vi "蝴蝶图 copy.vi"() -> ()   [LabVIEW 2023]
panel:
  out "XY Graph":cluster{"Y":dbl[], "Y":dbl[]}[](graph)
  out "return value":dbl[][](array[numeric])
  in  "Array 3":dbl[][](array[numeric])
  in  "module path 2":path
  out "error out 2":errorcluster
  out "error out":errorcluster
  in  "module path":path
  out "Array 2":string[](array[string])
  in  "String":string
  in  "Array":string[](array[string])
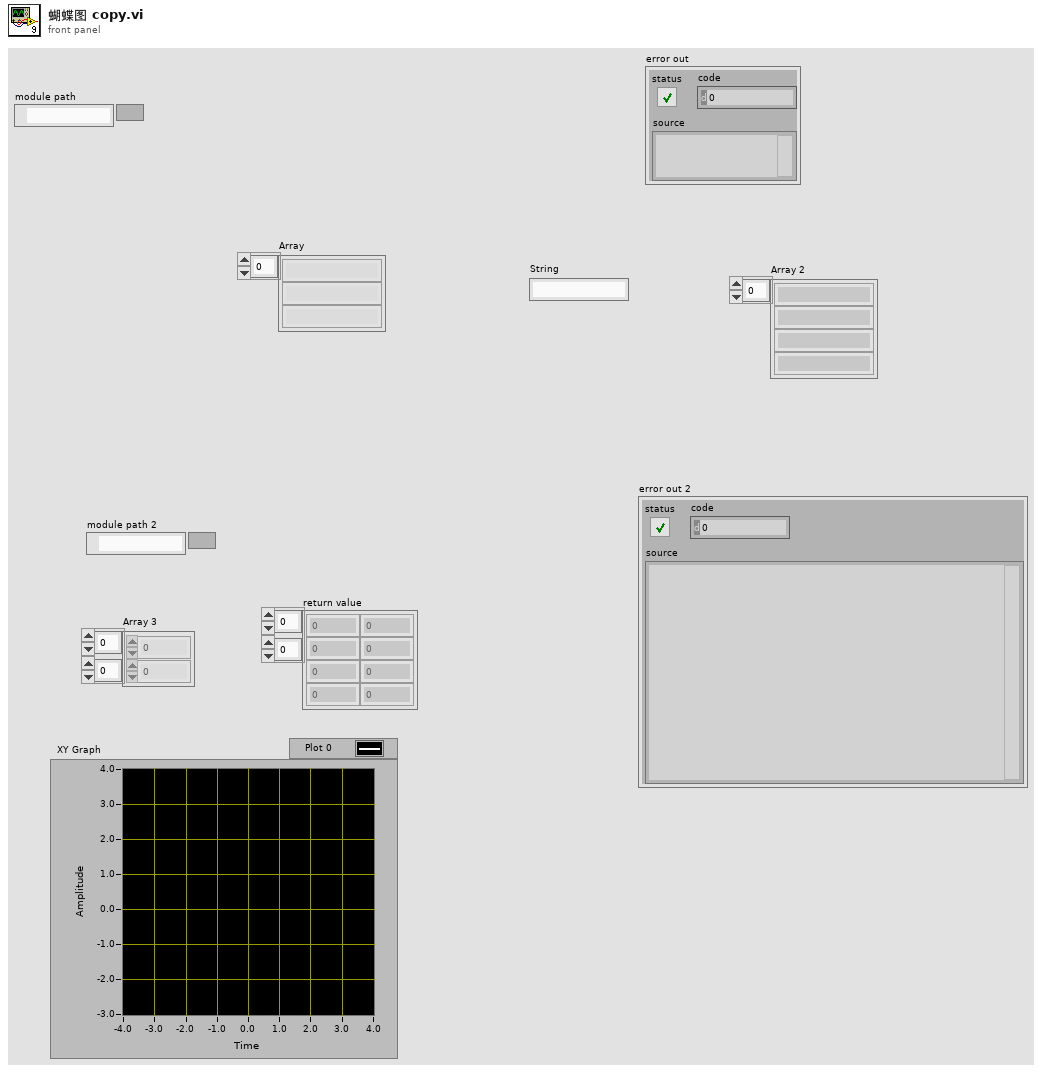
[diagram p1: front panel]
types:
  T1 = typedef "imagedata.ctl" = cluster{"image type":i32, "image depth":i32, "image":u8[], "mask":u8[], "colors":u32[], "Rectangle":cluster{"left":i16, "top":i16, "right":i16, "bottom":i16}}
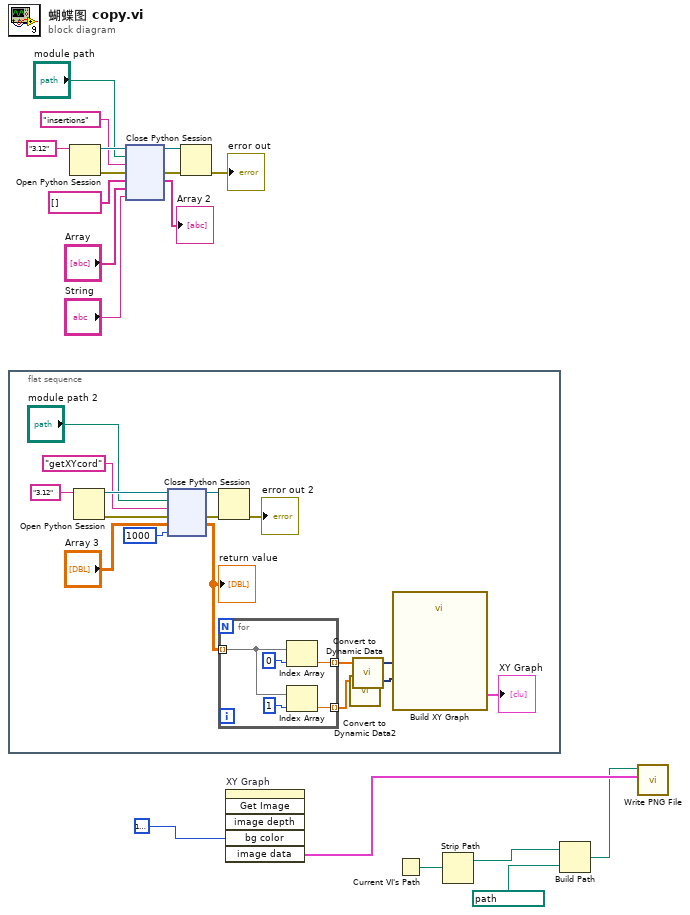
[diagram p0: block diagram]
diagram:
  n1 = flat-sequence {
    frame #0 {
      n2 = Open Python Session(python version="3.12" ("Python version")) -> (session out=w34:refnum<k35>, error out=w32:errorcluster)  [unwired: 2 in]
      n3 = node(w34, "module path 2", "getXYcord" ("function name"), w32, "Array 3", 1000) -> (w33:refnum<k35>, w31:errorcluster, w24:dbl[][])  [unwired: 1 in, 2 out]
      "return value" <- w24
      n4 = Close Python Session(session in=w33, error in=w31) -> (11:→"error out 2":errorcluster)
      n5 = for {
        tunnel: w24 -> [w38] mode=indexing
        tunnel: [w36] -> w22 mode=indexing
        tunnel: [w35] -> w20 mode=indexing
        n6 = Index Array(array=w38, index=0) -> (element=w36:dbl)
        n7 = Index Array(array=w38, index=1) -> (element=w35:dbl)
      }
      n8 = call "Convert to Dynamic Data2"("Array"=w20) -> ("Dynamic Data Type"=w19:dynamicdata)  [unwired: 3 in]
      n9 = call "Convert to Dynamic Data"("Array"=w22) -> ("Dynamic Data Type"=w21:dynamicdata)  [unwired: 3 in]
      n10 = call "Build XY Graph"("Y Input"=w19, "X Input"=w21) -> ("XY Graph"=→"XY Graph":cluster{"X":dbl[], "Y":dbl[]}[])  [unwired: 8 in, 1 out]
    }
  }
  n11 = Open Python Session(python version="3.12" ("Python version")) -> (session out=w17:refnum<k35>, error out=w13:errorcluster)  [unwired: 2 in]
  n12 = node(w17, "module path", "insertions" ("function name"), w13, string[] [], "Array", "String") -> (w15:refnum<k35>, w14:errorcluster, →"Array 2":string[])  [unwired: 2 in, 2 out]
  n13 = Close Python Session(session in=w15, error in=w14) -> (11:→"error out":errorcluster)
  n14 = invoke on="XY Graph" class="XYGraph (strict)" method="Get Image"("bg color"=u32 16777238) -> ("image data"=w5:T1)  [unwired: 5 in, 5 out]
  n15 = Current VI's Path() -> (path=w4:path)
  n16 = Strip Path(path=w4) -> (stripped path=w3:path)  [unwired: 1 out]
  n17 = Build Path(base path=w3, name or relative path=path "蝴蝶图.png") -> (appended path=w1:path)
  n18 = call <vilib>:"Write PNG File.vi"("image data"=w5, "path to PNG file"=w1) -> ()  [unwired: 8 in, 2 out]
